vi "Sony LANC remote.vi"() -> ()   [LabVIEW 2022 SP3]
panel:
  in  "plus":bool
  in  "minus":bool
  in  "15key":bool
  in  "16key":bool
  in  "7key":bool
  in  "8key":bool
  in  "9key":bool
  in  "10key":bool
  in  "11key":bool
  in  "12key":bool
  in  "13key":bool
  in  "14key":bool
  in  "1key":bool caption="Keypad"
  in  "2key":bool
  in  "3key":bool
  in  "4key":bool
  in  "5key":bool
  in  "6key":bool
  in  "EEPROM_store":bool
  in  "EEPROM_read":bool
  in  "valup":bool caption="Data"
  in  "valdn":bool
  in  "adup":bool caption="Addr"
  in  "addn":bool
  in  "pgup":bool caption="Page"
  in  "pgdn":bool
  out "EEPROM":string
  in  "send_custom":bool
  in  "eject":bool
  in  "fwd":bool
  in  "rew":bool
  in  "stop":bool
  in  "pause":bool
  in  "play":bool
  in  "enter":bool
  in  "menu":bool
  in  "right":bool
  in  "left":bool
  in  "up":bool
  in  "down":bool
  in  "Command":string(combo)
  out "Time":string
  out "Date":string
  out "data_code":cluster{"year/hour":u32, "month/min":u32}
  out "data_type":u8(ring) items=["Undefined"=0, "Date"=3, "Time"=4]
  out "Remaining time":string
  out "Real time counter":string
  out "RCTC":bool
  out "min_sec":cluster{"min":u32, "sec":u32}
  out "Decimal counter":u32
  out "Features":T1 {"Capability" items=["V8"=0, "DV"=1, "DV"=2, "Hi8"=4]; "Input" items=["Tuner"=0, "Sim."=1, "Line"=3]; "Thickness" items=["10µm", "13µm"]; "Type" items=["MP", "ME"]; "Speed" items=["SP", "LP"]}
  out "Status":string
  out "EOP":bool
  in  "stop":bool
  in  "send":bool
  in  "cmd":string caption="Custom cmd (2 bytes hex)"
  # "Tape"
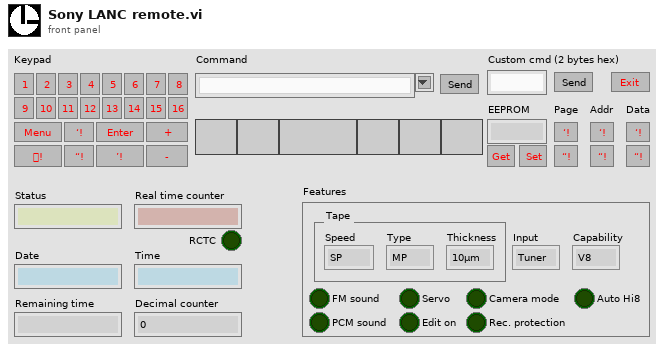
[diagram p1: front panel]
types:
  T1 = cluster{"Speed":u8, "FM sound":bool, "PCM sound":bool, "Camera mode":bool, "Rec. protection":bool, "Type":u8, "Thickness":u8, "Servo":bool, "Input":u8, "Capability":u8, "Edit on":bool, "Auto Hi8":bool}
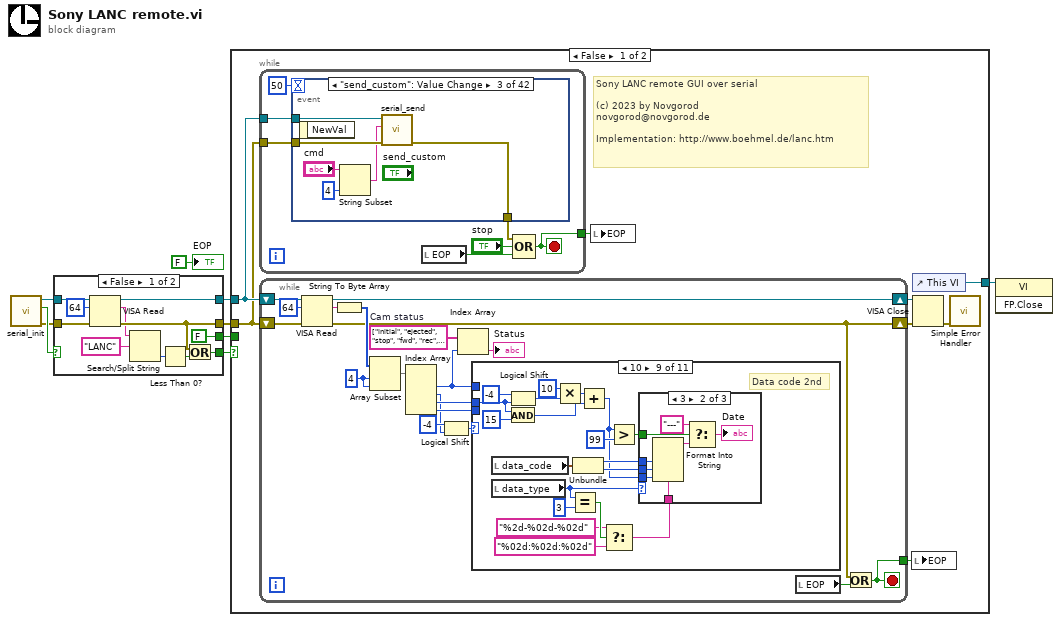
[diagram p0: block diagram]
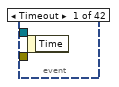
[diagram p3: hidden frame]
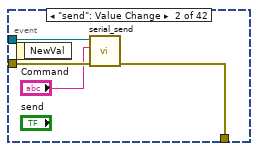
[diagram p4: hidden frame]
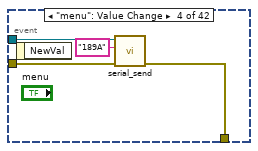
[diagram p5: hidden frame]
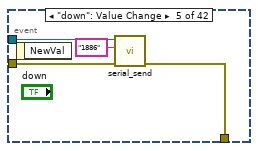
[diagram p6: hidden frame]
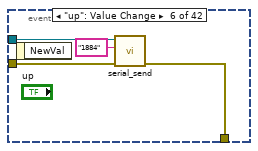
[diagram p7: hidden frame]
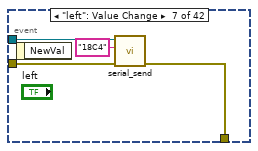
[diagram p8: hidden frame]
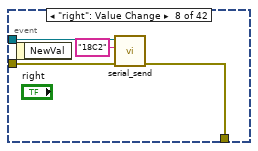
[diagram p9: hidden frame]
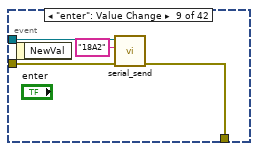
[diagram p10: hidden frame]
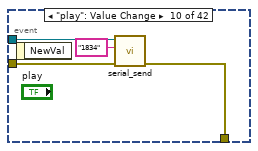
[diagram p11: hidden frame]
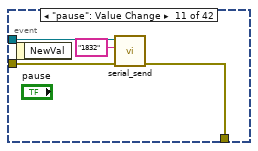
[diagram p12: hidden frame]
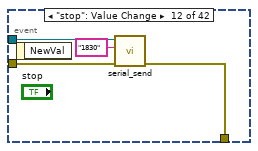
[diagram p13: hidden frame]
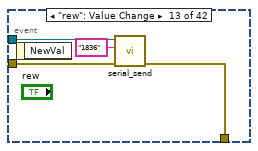
[diagram p14: hidden frame]
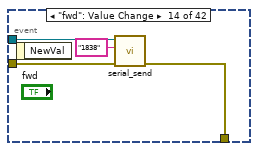
[diagram p15: hidden frame]
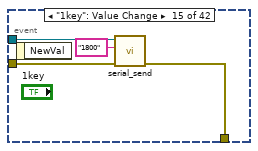
[diagram p16: hidden frame]
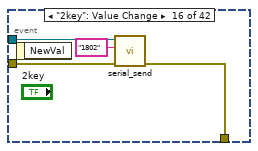
[diagram p17: hidden frame]
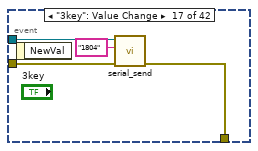
[diagram p18: hidden frame]
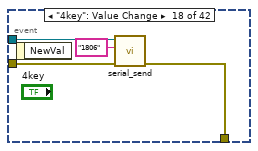
[diagram p19: hidden frame]
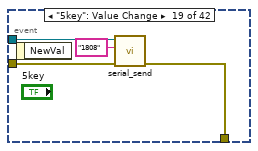
[diagram p20: hidden frame]
diagram:
  n1 = call "serial_init.vi"() -> ("error out"=w3:errorcluster, "Cancelled?"=w4:bool, "VISA out"=w5:refnum<visa-resource-name>)  [unwired: 9 in]
  n2 = case shown="False" w4 {
    selector: w4 -> [_ w21]
    tunnel: [w20 w22] -> w9
    tunnel: [w19 _] -> w8
    tunnel: [w18 w21] -> w7
    tunnel: w5 -> [w12 w22]
    tunnel: w3 -> [w11 _]
    tunnel: [FALSE w21] -> w1
    frame False {
      n3 = VISA Read(VISA resource name=w12, byte count=u32 64, error in (no error)=w11) -> (VISA resource name out=w20:refnum<visa-resource-name>, read buffer=w16:string, error out=w19:errorcluster)  [unwired: 1 out]
      n4 = Search/Split String(string=w16, search string/char (-)="LANC") -> (offset of match=w14:i32)  [unwired: 1 in, 2 out]
      n5 = Less Than 0?(x=w14) -> (x < 0?=w13:bool)
      n6 = Or(x=w19, y=w13) -> (x .or. y?=w18:bool)
    }
    frame True {
    }
  }
  n7 = case shown="False" w7 {
    tunnel: w9 -> [w27 w402]
    tunnel: w8 -> [w26 _]
    tunnel: [w23 w403] -> w2
    tunnel: w1 -> [_ w401]
    frame False {
      # "Sony LANC remote GUI over serial\n\n(c) 2023 by Novgorod\nnovgorod@novgorod.de\n\nImplementation: http://www.boehmel.de/lanc.htm"
      n8 = while {
        tunnel: w26 -> [w35]
        tunnel: w27 -> [w36]
        tunnel: [w32] -> w24
        stop <- w32 stop-if-true
        n9 = event shown="[2] \"send_custom\": Value Change" {
          selector: _ -> [_ _ _ _ _ _ _ _ _ _ _ _ _ _ _ _ _ _ _ _ _ _ _ _ _ _ _ _ _ _ _ _ _ _ _ _ _ _ _ _ _ _]
          dyn-events: _ -> [_ _ _ _ _ _ _ _ _ _ _ _ _ _ _ _ _ _ _ _ _ _ _ _ _ _ _ _ _ _ _ _ _ _ _ _ _ _ _ _ _ _]
          timeout: 50 -> [_ _ _ _ _ _ _ _ _ _ _ _ _ _ _ _ _ _ _ _ _ _ _ _ _ _ _ _ _ _ _ _ _ _ _ _ _ _ _ _ _ _]
          tunnel: w36 -> [_ w41 w47 w51 w55 w59 w63 w67 w71 w75 w79 w83 w87 w91 w95 w99 w103 w107 w111 w115 w119 w123 w127 w131 w135 w139 w143 w147 w151 w155 w159 w163 w168 w177 w181 w185 w189 w193 w197 w201 w205 _]
          tunnel: w35 -> [_ w40 w46 w50 w54 w58 w62 w66 w70 w74 w78 w82 w86 w90 w94 w98 w102 w106 w110 w114 w118 w122 w126 w130 w134 w138 w142 w146 w150 w154 w158 w162 w167 w176 w180 w184 w188 w192 w196 w200 w204 _]
          tunnel: [_ w39 w45 w49 w53 w57 w61 w65 w69 w73 w77 w81 w85 w89 w93 w97 w101 w105 w109 w113 w117 w121 w125 w129 w133 w137 w141 w145 w149 w153 w157 w161 w166 w175 w179 w183 w187 w191 w195 w199 w203 errorcluster {"status"=TRUE, "code"=0, "source"=""} ("error out")] -> w34
          event Timeout {
            n10 = event-data() -> ()  [unwired: 1 in, 1 out]
          }
          event "send": Value Change {
            n11 = event-data() -> ()  [unwired: 1 in, 1 out]
            n12 = call "serial_send.vi"("error in (no error)"=w40, "Send buffer"="Command", "VISA in"=w41) -> ("error out"=w39:errorcluster)  [unwired: 7 in, 1 out]
          }
          event "send_custom": Value Change {
            n13 = event-data() -> ()  [unwired: 1 in, 1 out]
            n14 = String Subset(string="cmd", length (rest)=4 ("length (rest)")) -> (substring=w42:string)  [unwired: 1 in]
            n15 = call "serial_send.vi"("error in (no error)"=w46, "Send buffer"=w42, "VISA in"=w47) -> ("error out"=w45:errorcluster)  [unwired: 7 in, 1 out]
          }
          event "menu": Value Change {
            n16 = event-data() -> ()  [unwired: 1 in, 1 out]
            n17 = call "serial_send.vi"("error in (no error)"=w50, "Send buffer"="189A", "VISA in"=w51) -> ("error out"=w49:errorcluster)  [unwired: 7 in, 1 out]
          }
          event "down": Value Change {
            n18 = event-data() -> ()  [unwired: 1 in, 1 out]
            n19 = call "serial_send.vi"("error in (no error)"=w54, "Send buffer"="1886", "VISA in"=w55) -> ("error out"=w53:errorcluster)  [unwired: 7 in, 1 out]
          }
          event "up": Value Change {
            n20 = event-data() -> ()  [unwired: 1 in, 1 out]
            n21 = call "serial_send.vi"("error in (no error)"=w58, "Send buffer"="1884", "VISA in"=w59) -> ("error out"=w57:errorcluster)  [unwired: 7 in, 1 out]
          }
          event "left": Value Change {
            n22 = event-data() -> ()  [unwired: 1 in, 1 out]
            n23 = call "serial_send.vi"("error in (no error)"=w62, "Send buffer"="18C4", "VISA in"=w63) -> ("error out"=w61:errorcluster)  [unwired: 7 in, 1 out]
          }
          event "right": Value Change {
            n24 = event-data() -> ()  [unwired: 1 in, 1 out]
            n25 = call "serial_send.vi"("error in (no error)"=w66, "Send buffer"="18C2", "VISA in"=w67) -> ("error out"=w65:errorcluster)  [unwired: 7 in, 1 out]
          }
          event "enter": Value Change {
            n26 = event-data() -> ()  [unwired: 1 in, 1 out]
            n27 = call "serial_send.vi"("error in (no error)"=w70, "Send buffer"="18A2", "VISA in"=w71) -> ("error out"=w69:errorcluster)  [unwired: 7 in, 1 out]
          }
          event "play": Value Change {
            n28 = event-data() -> ()  [unwired: 1 in, 1 out]
            n29 = call "serial_send.vi"("error in (no error)"=w74, "Send buffer"="1834", "VISA in"=w75) -> ("error out"=w73:errorcluster)  [unwired: 7 in, 1 out]
          }
          event "pause": Value Change {
            n30 = event-data() -> ()  [unwired: 1 in, 1 out]
            n31 = call "serial_send.vi"("error in (no error)"=w78, "Send buffer"="1832", "VISA in"=w79) -> ("error out"=w77:errorcluster)  [unwired: 7 in, 1 out]
          }
          event "stop": Value Change {
            n32 = event-data() -> ()  [unwired: 1 in, 1 out]
            n33 = call "serial_send.vi"("error in (no error)"=w82, "Send buffer"="1830", "VISA in"=w83) -> ("error out"=w81:errorcluster)  [unwired: 7 in, 1 out]
          }
          event "rew": Value Change {
            n34 = event-data() -> ()  [unwired: 1 in, 1 out]
            n35 = call "serial_send.vi"("error in (no error)"=w86, "Send buffer"="1836", "VISA in"=w87) -> ("error out"=w85:errorcluster)  [unwired: 7 in, 1 out]
          }
          event "fwd": Value Change {
            n36 = event-data() -> ()  [unwired: 1 in, 1 out]
            n37 = call "serial_send.vi"("error in (no error)"=w90, "Send buffer"="1838", "VISA in"=w91) -> ("error out"=w89:errorcluster)  [unwired: 7 in, 1 out]
          }
          event "1key": Value Change {
            n38 = event-data() -> ()  [unwired: 1 in, 1 out]
            n39 = call "serial_send.vi"("error in (no error)"=w94, "Send buffer"="1800", "VISA in"=w95) -> ("error out"=w93:errorcluster)  [unwired: 7 in, 1 out]
          }
          event "2key": Value Change {
            n40 = event-data() -> ()  [unwired: 1 in, 1 out]
            n41 = call "serial_send.vi"("error in (no error)"=w98, "Send buffer"="1802", "VISA in"=w99) -> ("error out"=w97:errorcluster)  [unwired: 7 in, 1 out]
          }
          event "3key": Value Change {
            n42 = event-data() -> ()  [unwired: 1 in, 1 out]
            n43 = call "serial_send.vi"("error in (no error)"=w102, "Send buffer"="1804", "VISA in"=w103) -> ("error out"=w101:errorcluster)  [unwired: 7 in, 1 out]
          }
          event "4key": Value Change {
            n44 = event-data() -> ()  [unwired: 1 in, 1 out]
            n45 = call "serial_send.vi"("error in (no error)"=w106, "Send buffer"="1806", "VISA in"=w107) -> ("error out"=w105:errorcluster)  [unwired: 7 in, 1 out]
          }
          event "5key": Value Change {
            n46 = event-data() -> ()  [unwired: 1 in, 1 out]
            n47 = call "serial_send.vi"("error in (no error)"=w110, "Send buffer"="1808", "VISA in"=w111) -> ("error out"=w109:errorcluster)  [unwired: 7 in, 1 out]
          }
          event "6key": Value Change {
            n48 = event-data() -> ()  [unwired: 1 in, 1 out]
            n49 = call "serial_send.vi"("error in (no error)"=w114, "Send buffer"="180A", "VISA in"=w115) -> ("error out"=w113:errorcluster)  [unwired: 7 in, 1 out]
          }
          event "7key": Value Change {
            n50 = event-data() -> ()  [unwired: 1 in, 1 out]
            n51 = call "serial_send.vi"("error in (no error)"=w118, "Send buffer"="180C", "VISA in"=w119) -> ("error out"=w117:errorcluster)  [unwired: 7 in, 1 out]
          }
          event "8key": Value Change {
            n52 = event-data() -> ()  [unwired: 1 in, 1 out]
            n53 = call "serial_send.vi"("error in (no error)"=w122, "Send buffer"="180E", "VISA in"=w123) -> ("error out"=w121:errorcluster)  [unwired: 7 in, 1 out]
          }
          event "9key": Value Change {
            n54 = event-data() -> ()  [unwired: 1 in, 1 out]
            n55 = call "serial_send.vi"("error in (no error)"=w126, "Send buffer"="1810", "VISA in"=w127) -> ("error out"=w125:errorcluster)  [unwired: 7 in, 1 out]
          }
          event "10key": Value Change {
            n56 = event-data() -> ()  [unwired: 1 in, 1 out]
            n57 = call "serial_send.vi"("error in (no error)"=w130, "Send buffer"="1812", "VISA in"=w131) -> ("error out"=w129:errorcluster)  [unwired: 7 in, 1 out]
          }
          event "11key": Value Change {
            n58 = event-data() -> ()  [unwired: 1 in, 1 out]
            n59 = call "serial_send.vi"("error in (no error)"=w134, "Send buffer"="1814", "VISA in"=w135) -> ("error out"=w133:errorcluster)  [unwired: 7 in, 1 out]
          }
          event "12key": Value Change {
            n60 = event-data() -> ()  [unwired: 1 in, 1 out]
            n61 = call "serial_send.vi"("error in (no error)"=w138, "Send buffer"="1816", "VISA in"=w139) -> ("error out"=w137:errorcluster)  [unwired: 7 in, 1 out]
          }
          event "13key": Value Change {
            n62 = event-data() -> ()  [unwired: 1 in, 1 out]
            n63 = call "serial_send.vi"("error in (no error)"=w142, "Send buffer"="1818", "VISA in"=w143) -> ("error out"=w141:errorcluster)  [unwired: 7 in, 1 out]
          }
          event "14key": Value Change {
            n64 = event-data() -> ()  [unwired: 1 in, 1 out]
            n65 = call "serial_send.vi"("error in (no error)"=w146, "Send buffer"="181A", "VISA in"=w147) -> ("error out"=w145:errorcluster)  [unwired: 7 in, 1 out]
          }
          event "15key": Value Change {
            n66 = event-data() -> ()  [unwired: 1 in, 1 out]
            n67 = call "serial_send.vi"("error in (no error)"=w150, "Send buffer"="181C", "VISA in"=w151) -> ("error out"=w149:errorcluster)  [unwired: 7 in, 1 out]
          }
          event "16key": Value Change {
            n68 = event-data() -> ()  [unwired: 1 in, 1 out]
            n69 = call "serial_send.vi"("error in (no error)"=w154, "Send buffer"="181E", "VISA in"=w155) -> ("error out"=w153:errorcluster)  [unwired: 7 in, 1 out]
          }
          event "plus": Value Change {
            n70 = event-data() -> ()  [unwired: 1 in, 1 out]
            n71 = call "serial_send.vi"("error in (no error)"=w158, "Send buffer"="1820", "VISA in"=w159) -> ("error out"=w157:errorcluster)  [unwired: 7 in, 1 out]
          }
          event "minus": Value Change {
            n72 = event-data() -> ()  [unwired: 1 in, 1 out]
            n73 = call "serial_send.vi"("error in (no error)"=w162, "Send buffer"="1822", "VISA in"=w163) -> ("error out"=w161:errorcluster)  [unwired: 7 in, 1 out]
          }
          event "eject": Value Change {
            n74 = event-data() -> ()  [unwired: 1 in, 1 out]
            n75 = Two Button Dialog(message="Eject tape?") -> (T button?=w164:bool)  [unwired: 2 in]
            n76 = case shown="True" w164 {
              tunnel: w168 -> [_ w173]
              tunnel: w167 -> [w169 w172]
              tunnel: [w169 w171] -> w166
              frame False {
              }
              frame True {
                n77 = call "serial_send.vi"("error in (no error)"=w172, "Send buffer"="182C", "VISA in"=w173) -> ("error out"=w171:errorcluster)  [unwired: 7 in, 1 out]
              }
            }
          }
          event "EEPROM_read": Value Change {
            n78 = event-data() -> ()  [unwired: 1 in, 1 out]
            n79 = call "serial_send.vi"("error in (no error)"=w176, "Send buffer"="FF00", "VISA in"=w177) -> ("error out"=w175:errorcluster)  [unwired: 7 in, 1 out]
          }
          event "EEPROM_store": Value Change {
            n80 = event-data() -> ()  [unwired: 1 in, 1 out]
            n81 = call "serial_send.vi"("error in (no error)"=w180, "Send buffer"="FF32", "VISA in"=w181) -> ("error out"=w179:errorcluster)  [unwired: 7 in, 1 out]
          }
          event "pgup": Value Change {
            n82 = event-data() -> ()  [unwired: 1 in, 1 out]
            n83 = call "serial_send.vi"("error in (no error)"=w184, "Send buffer"="FF67", "VISA in"=w185) -> ("error out"=w183:errorcluster)  [unwired: 7 in, 1 out]
          }
          event "pgdn": Value Change {
            n84 = event-data() -> ()  [unwired: 1 in, 1 out]
            n85 = call "serial_send.vi"("error in (no error)"=w188, "Send buffer"="FF65", "VISA in"=w189) -> ("error out"=w187:errorcluster)  [unwired: 7 in, 1 out]
          }
          event "adup": Value Change {
            n86 = event-data() -> ()  [unwired: 1 in, 1 out]
            n87 = call "serial_send.vi"("error in (no error)"=w192, "Send buffer"="FF38", "VISA in"=w193) -> ("error out"=w191:errorcluster)  [unwired: 7 in, 1 out]
          }
          event "addn": Value Change {
            n88 = event-data() -> ()  [unwired: 1 in, 1 out]
            n89 = call "serial_send.vi"("error in (no error)"=w196, "Send buffer"="FF36", "VISA in"=w197) -> ("error out"=w195:errorcluster)  [unwired: 7 in, 1 out]
          }
          event "valup": Value Change {
            n90 = event-data() -> ()  [unwired: 1 in, 1 out]
            n91 = call "serial_send.vi"("error in (no error)"=w200, "Send buffer"="FF34", "VISA in"=w201) -> ("error out"=w199:errorcluster)  [unwired: 7 in, 1 out]
          }
          event "valdn": Value Change {
            n92 = event-data() -> ()  [unwired: 1 in, 1 out]
            n93 = call "serial_send.vi"("error in (no error)"=w204, "Send buffer"="FF30", "VISA in"=w205) -> ("error out"=w203:errorcluster)  [unwired: 7 in, 1 out]
          }
          event Panel Close? {
            n94 = event-data() -> ()  [unwired: 1 in, 1 out]
            n95 = event-data("Discard?"=TRUE) -> ()  [unwired: 1 in, 1 out]
          }
        }
        n96 = local read "EOP"() -> (w31:bool)
        n97 = Compound Arithmetic op=OR(w34, "stop", w31) -> (w32:bool)
      }
      n98 = while {
        shift-right: [w224] -> w29
        shift-left: w27 -> [w226]
        shift-right: [w219] -> w30
        shift-left: w26 -> [w225]
        tunnel: [w208] -> w25
        stop <- w208 stop-if-true
        w216 = string[] ["initial", "ejected", "stop", "fwd", "rec", "", "play", "play/pause fwd", "AL insert", "", "", "", "", "", "", "page 0", "", "dew cass. out", "laod", "", "rec/pause", "", "", "frame fwd", "AL ins-pause", "", "", "", "", "", "", "page 1", "", "ejecting", "cassette busy", "", "timer-rec", "", "x1 fwd", "1/5 fwd", "AR insert", "", "", "", "", "", "", "page 2", "", "unload", "low-battery", "go zero/play f.", "timer-rec s.", "", "x1 rev", "1/5 rev", "AR ins-pause", "", "", "", "", "", "", "page 3", "", "", "dew stop", "fwd mem stop", "AV insert", "", "cue", "1/10 fwd", "AL+V insert", "", "", "", "", "", "", "page 4", "", "", "emergency", "", "AV ins.-pause", "", "rev", "1/10 rev", "AL+V ins-ps", "", "", "", "", "", "", "page 5", "", "", "tape end", "", "video insert", "", "x2/x3 fwd", "frame fwd", "AR+V insert", "", "", "", "", "", "", "page 6", "", "", "tape top", "", "video ins.-ps", "", "x2/x3 rev", "frame rev", "AL+R ins-ps", "", "", "", "", "", "", "page 7", "", "", "", "rew", "audio dub", "edit search+", "x9 fwd", "", "", "", "", "", "", "", "", "page 8", "", "", "stp after zero", "", "a. dub pause", "edit search-", "x9 rev", "play/pause rev", "", "", "", "", "", "", "", "page 9", "", "", "load emer.", "auto-play", "cam rec", "edit-s fwd", "frame sea. cue", "", "", "", "", "", "", "", "", "page A", "", "unload emerg.", "stop emerg. 1", "go zero/play r.", "cam stby", "edit-s rev", "frame sea. rev", "", "", "", "", "", "", "", "", "page B", "", "", "stop emerg. 2", "rew mem stop", "", "", "x14 fwd", "", "", "", "", "", "", "", "", "page C", "", "", "", "hi-speed rew", "", "", "x14 rev", "", "", "", "", "", "", "", "", "page D", "", "", "stop NC", "", "", "", "", "", "", "", "", "", "", "", "", "page E", "", "", "", "", "", "edit pause", "", "", "", "", "", "", "", "", "", "page F"]  # Cam status
        w218 = 4 ("index")
        n99 = VISA Read(VISA resource name=w226, byte count=u32 64, error in (no error)=w225) -> (VISA resource name out=w224:refnum<visa-resource-name>, read buffer=w222:string, error out=w219:errorcluster)  [unwired: 1 out]
        n100 = String To Byte Array(string=w222) -> (unsigned byte array=w221:u8[])
        n101 = Array Subset(array=w221, index=w218, length=w218) -> (w217:u8[])
        n102 = Index Array(array=w217) -> (element #1=w209:u8, element #2=w210:u8, element #3=w211:u8, element #4=w212:u8)  [unwired: 4 in]
        n103 = Logical Shift(y=i16 -4, x=w210) -> (x << y=w213:u8)
        n104 = Index Array(array=w216, index=w209) -> (element=→"Status":string)
        n105 = case shown="10" w213 {
          tunnel: w212 -> [_ w249 w262 w279 w306 w328 w331 w343 _ w388 w395]
          tunnel: w211 -> [_ w250 w263 w280 w314 w329 _ w344 w365 w392 w396]
          tunnel: w209 -> [_ _ _ _ _ _ _ _ _ _ w400]
          frame 0, Default {
          }
          frame 1 {
            # "Status V8 and Hi8"
            n106 = Join Numbers(hi=w249, lo=w250) -> ((hi.lo)=w248:u16)
            n107 = Number To Boolean Array(number=w248) -> (Boolean array=w247:bool[])
            n108 = Index Array(array=w247, index #2=2 ("index"), index #8=11 ("index"), index #10=14 ("index")) -> (element #1=w246:bool, element #2=w235:bool, element #3=w234:bool, element #4=w233:bool, element #5=w232:bool, element #6=w244:bool, element #7=w243:bool, element #8=w229:bool, element #9=w241:bool, element #10=w239:bool)  [unwired: 7 in]
            n109 = Boolean To (0,1)(Boolean=w246) -> (0, 1=w236:i16)
            n110 = Boolean To (0,1)(Boolean=w244) -> (0, 1=w231:i16)
            n111 = Boolean To (0,1)(Boolean=w243) -> (0, 1=w230:i16)
            n112 = Build Array(w241, w239) -> (w238:bool[])
            n113 = local read "Features"() -> (w237:T1)
            n114 = Boolean Array To Number(Boolean array=w238) -> (number=w228:u32)
            n115 = Bundle(cluster=w237, "Speed"=w236, "FM sound"=w235, "PCM sound"=w234, "Camera mode"=w233, "Rec. protection"=w232, "Type"=w231, "Thickness"=w230, "Servo"=w229, "Input"=w228) -> (→"Features":T1)  [unwired: 3 in]
          }
          frame 2 {
            # "Decimal counter"
            n116 = Logical Shift(y=i16 -4, x=w262) -> (x << y=w258:u8)
            n117 = And(x=w262, y=u8 15) -> (x .and. y?=w256:u8)
            n118 = Logical Shift(y=i16 -4, x=w263) -> (x << y=w261:u8)
            n119 = And(x=w263, y=u8 15) -> (x .and. y?=w254:u8)
            n120 = Multiply(x=u32 10, y=w261) -> (x*y=w255:u32)
            n121 = Multiply(x=u32 1000, y=w258) -> (x*y=w253:u32)
            n122 = Multiply(x=u32 100, y=w256) -> (x*y=w252:u32)
            n123 = Compound Arithmetic op=ADD(w255, w254, w253, w252) -> (→"Decimal counter":u32)
          }
          frame 3 {
            # "Real time counter 1st"
            n124 = Logical Shift(y=i16 -4, x=w279) -> (x << y=w275:u8)
            n125 = And(x=w279, y=u8 15) -> (x .and. y?=w271:u8)
            n126 = Logical Shift(y=i16 -4, x=w280) -> (x << y=w278:u8)
            n127 = And(x=w280, y=u8 15) -> (x .and. y?=w273:u8)
            n128 = Multiply(x=u32 10, y=w278) -> (x*y=w274:u32)
            n129 = Multiply(x=u32 10, y=w275) -> (x*y=w272:u32)
            n130 = Add(x=w274, y=w273) -> (x+y=w269:u32)
            n131 = Add(x=w272, y=w271) -> (x+y=w270:u32)
            n132 = Bundle(w270, w269) -> (→"min_sec":cluster{u32, u32})  [unwired: 1 in]
          }
          frame 4 {
            # "Real time counter 2nd"
            n133 = Number To Boolean Array(number=w306) -> (Boolean array=w305:bool[])
            n134 = Logical Shift(y=i16 -4, x=w306) -> (x << y=w293:u8)
            n135 = And(x=w306, y=u8 15) -> (x .and. y?=w307:u8)
            n136 = Logical Shift(y=i16 -4, x=w314) -> (x << y=w313:u8)
            n137 = And(x=w314, y=u8 15) -> (x .and. y?=w309:u8)
            n138 = Index Array(array=w305, index #1=6 ("index")) -> (element #1=→"RCTC":bool, element #2=w302:bool)  [unwired: 1 in]
            n139 = local read "min_sec"() -> (w296:cluster{"min":u32, "sec":u32})
            n140 = And(x=u8 3, y=w293) -> (x .and. y?=w291:u8)
            n141 = Multiply(x=u32 10, y=w313) -> (x*y=w310:u32)
            n142 = Add(x=w310, y=w309) -> (x+y=w290:u32)
            n143 = Multiply(x=u32 10, y=w291) -> (x*y=w308:u32)
            n144 = Select(t="-", s=w302, f="") -> (s? t:f=w299:string)
            n145 = Unbundle(w296) -> ("min"=w295:u32, "sec"=w294:u32)
            n146 = Add(x=w308, y=w307) -> (x+y=w297:u32)
            n147 = Greater?(x=w290, y=u32 99) -> (0:w288:bool)
            n148 = Format Into String(format string="%d:%02d:%02d:%02d", initial string=w299, w290, w295, w294, w297) -> (resulting string=w287:string)  [unwired: 1 in, 1 out]
            n149 = Select(t="---", s=w288, f=w287) -> (s? t:f=→"Real time counter":string)
          }
          frame 5 {
            w320 = u8 15
            # "Remaining time"
            n150 = Logical Shift(y=i16 -4, x=w329) -> (x << y=w327:u8)
            n151 = And(x=w329, y=w320) -> (x .and. y?=w324:u8)
            n152 = And(x=w328, y=w320) -> (x .and. y?=w321:u8)
            n153 = Multiply(x=u32 10, y=w327) -> (x*y=w325:u32)
            n154 = Add(x=w325, y=w324) -> (x+y=w322:u32)
            n155 = Format Into String(format string="%d:%02d", w321, w322) -> (resulting string=→"Remaining time":string)  [unwired: 2 in, 1 out]
          }
          frame 8 {
            # "Data code type"
            "data_type" <- w331
          }
          frame 9 {
            # "Data code 1st"
            n156 = Logical Shift(y=i16 -4, x=w343) -> (x << y=w339:u8)
            n157 = And(x=w343, y=u8 15) -> (x .and. y?=w335:u8)
            n158 = Logical Shift(y=i16 -4, x=w344) -> (x << y=w342:u8)
            n159 = And(x=w344, y=u8 15) -> (x .and. y?=w337:u8)
            n160 = Multiply(x=u32 10, y=w342) -> (x*y=w338:u32)
            n161 = Multiply(x=u32 10, y=w339) -> (x*y=w336:u32)
            n162 = Add(x=w338, y=w337) -> (x+y=w333:u32)
            n163 = Add(x=w336, y=w335) -> (x+y=w334:u32)
            n164 = Bundle(w333, w334) -> (→"data_code":cluster{u32, u32})  [unwired: 1 in]
          }
          frame 10 {
            # "Data code 2nd"
            n165 = local read "data_code"() -> (w360:cluster{"year/hour":u32, "month/min":u32})
            n166 = local read "data_type"() -> (w357:u8)
            n167 = Logical Shift(y=i16 -4, x=w365) -> (x << y=w364:u8)
            n168 = And(x=w365, y=u8 15) -> (x .and. y?=w361:u8)
            n169 = Multiply(x=u32 10, y=w364) -> (x*y=w362:u32)
            n170 = Equal?(x=w357, y=u8 3) -> (x = y?=w356:bool)
            n171 = Unbundle(w360) -> ("year/hour"=w359:u32, "month/min"=w358:u32)
            n172 = Add(x=w362, y=w361) -> (x+y=w350:u32)
            n173 = Select(t="%2d-%02d-%02d" ("format string"), s=w356, f="%02d:%02d:%02d" ("format string")) -> (s? t:f=w353:string)
            n174 = Greater?(x=w350, y=u32 99) -> (0:w349:bool)
            n175 = case shown="3" w357 {
              tunnel: w353 -> [_ w375 w383]
              tunnel: w350 -> [_ w374 w382]
              tunnel: w359 -> [_ w373 w381]
              tunnel: w358 -> [_ w372 w380]
              tunnel: w349 -> [_ w369 w378]
              frame 0, Default {
              }
              frame 3 {
                n176 = Format Into String(format string=w375, w373, w372, w374) -> (resulting string=w370:string)  [unwired: 2 in, 1 out]
                n177 = Select(t="---", s=w369, f=w370) -> (s? t:f=→"Date":string)
              }
              frame 4 {
                n178 = Format Into String(format string=w383, w381, w380, w382) -> (resulting string=w377:string)  [unwired: 2 in, 1 out]
                n179 = Select(t="---", s=w378, f=w377) -> (s? t:f=→"Time":string)
              }
            }
          }
          frame 12 {
            # "Status Hi8, DV"
            n180 = Number To Boolean Array(number=w388) -> (Boolean array=w387:bool[])
            n181 = And(x=w392, y=u8 15) -> (x .and. y?=w390:u8)
            n182 = Index Array(array=w387, index #1=2 ("index")) -> (element #1=w385:bool, element #2=w384:bool)  [unwired: 1 in]
            n183 = local read "Features"() -> (w391:T1)
            n184 = Bundle By Name(cluster=w391, "Capability"=w390, "Edit on"=w385, "Auto Hi8"=w384) -> (w389:T1)
            n185 = local write "Features"(w389) -> ()
          }
          frame 15 {
            # "EEPROM"
            n186 = Logical Shift(y=i16 -4, x=w400) -> (x << y=w397:u8)
            n187 = Format Into String(format string="%x:%02x:%02x", w397, w396, w395) -> (resulting string=→"EEPROM":string)  [unwired: 2 in, 1 out]
          }
        }
        n188 = local read "EOP"() -> (w220:bool)
        n189 = Or(x=w219, y=w220) -> (x .or. y?=w208:bool)
      }
      n190 = local write "EOP"(w24) -> ()
      n191 = local write "EOP"(w25) -> ()
      n192 = control-ref of="This VI"() -> (w23:refnum<vi>)
      n193 = VISA Close(VISA resource name=w29, error in (no error)=w30) -> (error out=w28:errorcluster)
      n194 = call <vilib>:"Simple Error Handler.vi"("error in (no error)"=w28) -> ()  [unwired: 4 in, 5 out]
    }
    frame True {
      n195 = case shown="False" w401 {
        tunnel: "LANC interface not found!" ("search string/char (-)") -> [w407 _]
        tunnel: w402 -> [w406 _]
        frame False {
          n196 = One Button Dialog(message=w407) -> ()  [unwired: 1 in, 1 out]
          n197 = VISA Close(VISA resource name=w406) -> (error out=w405:errorcluster)  [unwired: 1 in]
          n198 = call <vilib>:"Clear Errors.vi"("error in (no error)"=w405) -> ()  [unwired: 5 in, 2 out]
        }
        frame True {
        }
      }
      n199 = control-ref of="This VI"() -> (w403:refnum<vi>)
    }
  }
  n200 = invoke class="VI" method="FP.Close"(reference=w2) -> ()  [unwired: 2 in, 3 out]
  "EOP" <- FALSE ("EOP")
